vi "IQA information.vi"() -> ()   [LabVIEW 2016]
uses:
  Control/iqa data.ctl
  <vilib>/Utility/miscctls.llb/LVPointTypeDef.ctl
panel:
  out "Array 2":T1[](array[typedef])
  out "Array":T1[](array[typedef])
  # "ITEM CODE"
  # "INVOICE CODE"
  # "INVOICE DATE"
  # "BEFORE IQA"
  # "AFTER IQA"
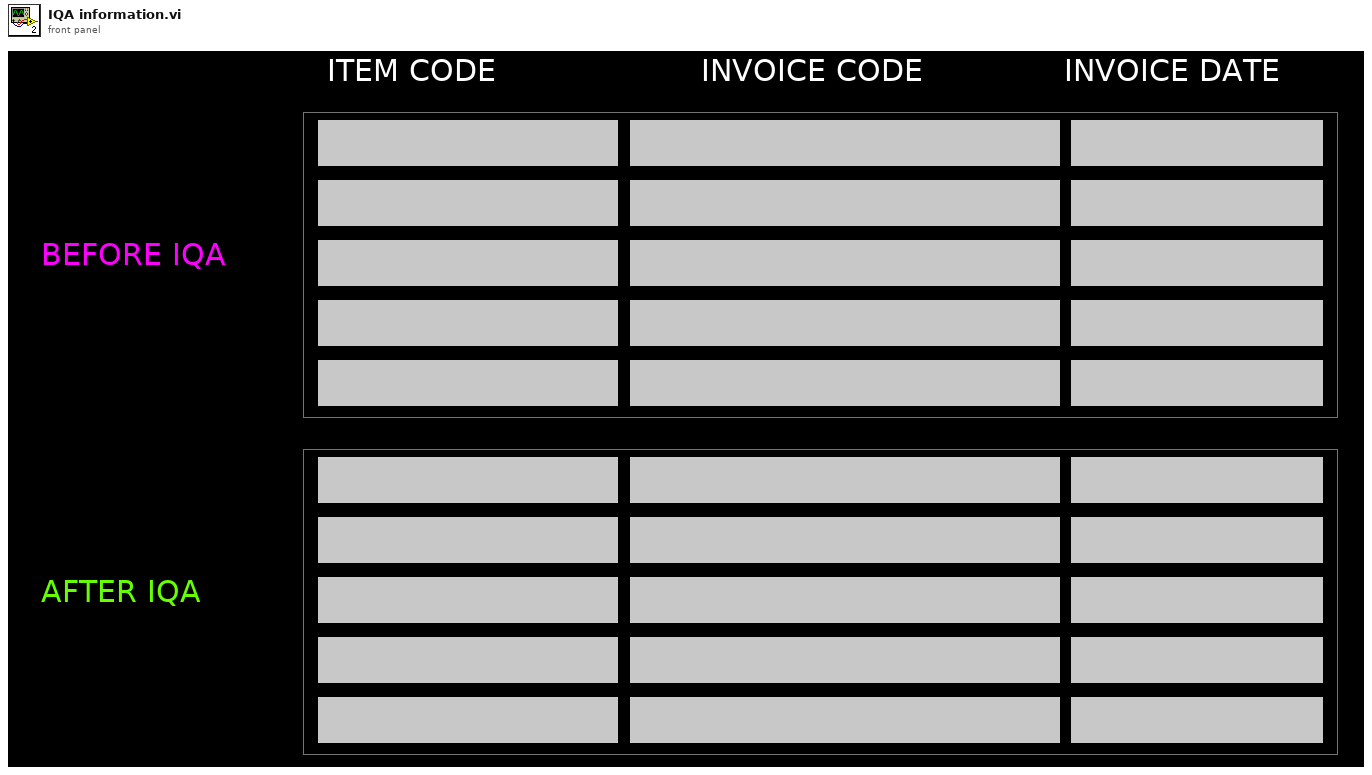
[diagram p1: front panel]
types:
  T1 = typedef "iqa data.ctl" = cluster{"ITEM CODE":string, "INVOICE CODE":string, "INVOICE DATE":string}
  T2 = typedef "LVPointTypeDef.ctl" = cluster{"Horizontal":i16, "Vertical":i16}
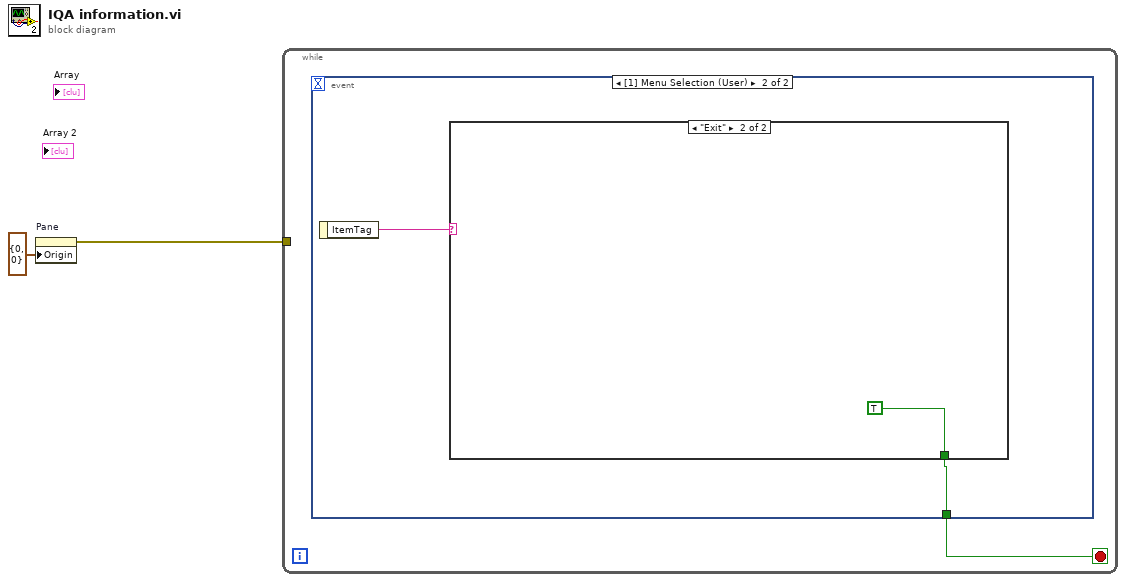
[diagram p0: block diagram]
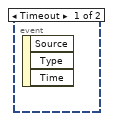
[diagram p2: hidden frame]
diagram:
  n1 = property on="Pane" class="Pane"("Origin"=T2 {"Horizontal"=0, "Vertical"=0}) -> (error out=w1:errorcluster)  [unwired: 2 in, 1 out]
  n2 = while {
    tunnel: w1 -> [_]
    stop <- w3 stop-if-true
    n3 = event shown="[1] Menu Selection (User)" {
      selector: _ -> [_ _]
      dyn-events: _ -> [_ _]
      timeout: _ -> [_ _]
      tunnel: [_ w4] -> w3
      event Timeout {
        n4 = event-data() -> ()  [unwired: 1 in, 3 out]
      }
      event Menu Selection (User) {
        n5 = event-data() -> ("ItemTag"=w5:string)  [unwired: 1 in]
        n6 = case shown="\"Exit\"" w5 {
          tunnel: [_ TRUE] -> w4
          frame "False", Default {
          }
          frame "Exit" {
          }
        }
      }
    }
  }
